vi "SubStage_WriteTableToExcel.vi"(7 "Record Table":string[][](table)=[["1", "09/01 17:55:24", "-0.7776", "0.4026", "Image", "green"], ["2", "09/01 17:55:35", "-1.7580", "-0.9129", "Image", "blue"], ["3", "09/01 17:55:42", "-2.7200", "0.4775", "Image", "yellow"]], 8 "error in (no error)":errorcluster, 10 "Completion Task":u16(ring) items=["Leave Excel Open", "Close Spreadsheet"], 11 "Path":path=path "C:/Users/ZouOptics/Desktop/ph.xlsx") -> (0 "error out":errorcluster)   [LabVIEW 2015]
doc: "This VI demonstrates the basic idea of using the OLE Automation VIs by writing a Table into an Excel WorkSheet."
panel:
  in  "row":i8=-1
  in  "column":i8=-1
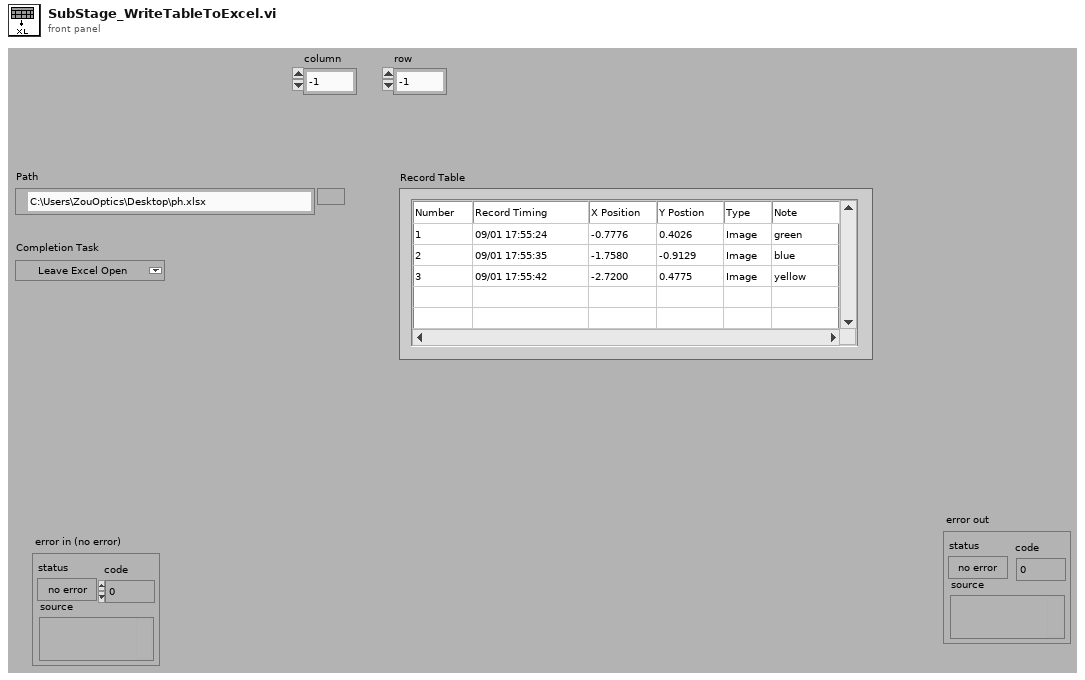
[diagram p1: front panel]
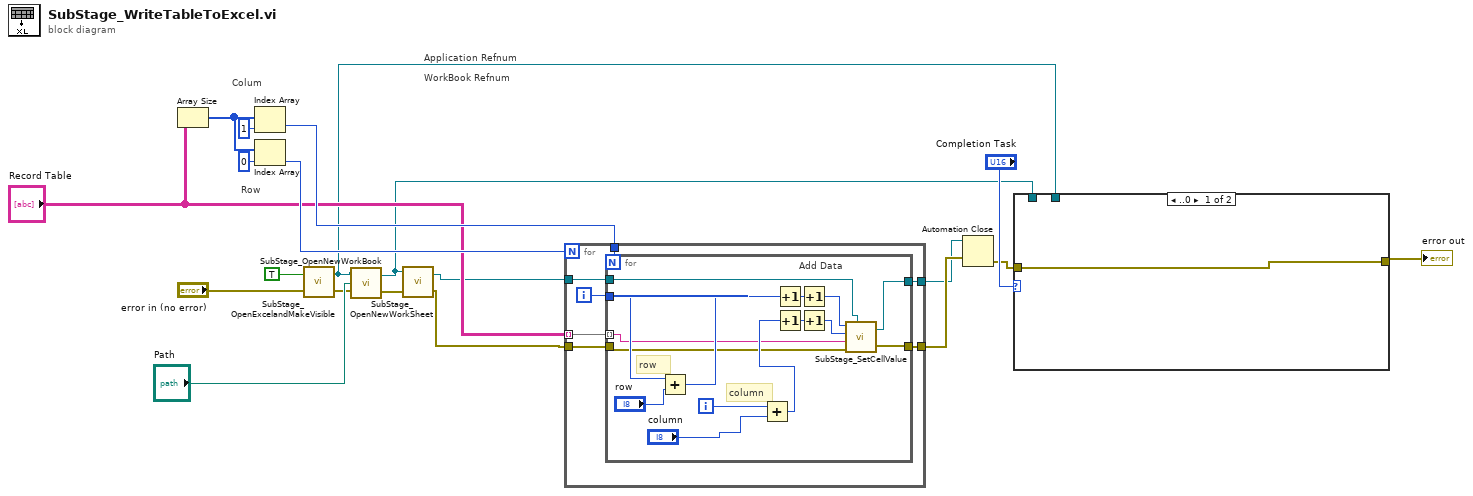
[diagram p0: block diagram]
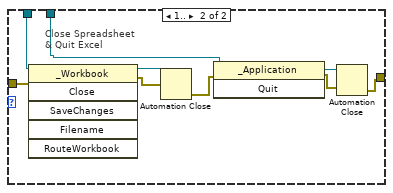
[diagram p2: hidden frame]
diagram:
  # "Colum"
  # "Row"
  # "WorkBook Refnum"
  # "Application Refnum"
  n1 = Array Size(array="Record Table") -> (size(s)=w20:i32[])
  n2 = Index Array(array=w20, index=1) -> (element=w17:i32)
  n3 = Index Array(array=w20, index=0) -> (element=w16:i32)
  n4 = call "SubStage_OpenExcelandMakeVisible.vi"("error in (no error)"="error in (no error)", "Visible Boolean"=TRUE) -> ("error out"=w5:errorcluster, "Excel._Application"=w7:refnum<k7>)
  n5 = call "SubStage_OpenNewWorkBook.vi"("error in (no error)"=w5, "File Path"="Path", "Excel._Application"=w7) -> ("error out"=w4:errorcluster, "Excel._Workbook"=w3:refnum<k7>)
  n6 = call "SubStage_OpenNewWorkSheet.vi"("error in (no error)"=w4, "Excel._Workbook"=w3) -> ("error out"=w2:errorcluster, "Excel._Worksheet"=w1:refnum<k7>)  [unwired: 1 in]
  n7 = for {
    N: w16 -> [_]
    tunnel: w1 -> [w27]
    tunnel: w2 -> [w24]
    tunnel: [w26] -> w13
    tunnel: "Record Table" -> [w23] mode=indexing
    tunnel: w17 -> [w22]
    tunnel: [w21] -> w11
    i -> [w25]
    n8 = for {
      N: w22 -> [_]
      tunnel: w27 -> [w30]
      tunnel: w24 -> [w34]
      tunnel: [w29] -> w26
      tunnel: w25 -> [w40]
      tunnel: w23 -> [w33] mode=indexing
      tunnel: [w28] -> w21
      i -> [w38]
      # "column"
      # "row"
      # "Add Data"
      n9 = Add(x=w40, y="row") -> (x+y=w39:i32)
      n10 = Add(x=w38, y="column") -> (x+y=w37:i32)
      n11 = Increment(x=w39) -> (x+1=w42:i32)
      n12 = Increment(x=w37) -> (x+1=w41:i32)
      n13 = Increment(x=w42) -> (x+1=w31:i32)
      n14 = Increment(x=w41) -> (x+1=w32:i32)
      n15 = call "SubStage_SetCellValue.vi"("Row"=w31, "Col"=w32, "Value"=w33, "error in (no error)"=w34, "Excel._Worksheet"=w30) -> ("Excel._Worksheet"=w28:refnum<k7>, "error out"=w29:errorcluster)
    }
  }
  n16 = Automation Close(3:w13, 5:w11) -> (0:w12:errorcluster)
  n17 = case shown="..0" "Completion Task" {
    tunnel: [w43 w44] -> w14
    tunnel: w3 -> [_ w52]
    tunnel: w7 -> [_ w48]
    tunnel: w12 -> [w43 w51]
    frame ..0 {
    }
    frame 1.. {
      # "Close Spreadsheet\n& Quit Excel"
      n18 = invoke class="_Workbook" method="Close"(reference=w52, error in=w51) -> (reference out=w50:refnum<k7>, error out=w49:errorcluster)  [unwired: 4 in, 4 out]
      n19 = Automation Close(3:w49, 5:w50) -> (0:w47:errorcluster)
      n20 = invoke class="_Application" method="Quit"(reference=w48, error in=w47) -> (reference out=w45:refnum<k7>, error out=w46:errorcluster)  [unwired: 1 in, 1 out]
      n21 = Automation Close(3:w46, 5:w45) -> (0:w44:errorcluster)
    }
  }
  "error out" <- w14
